vi "estimador de velocidades.vi"() -> (1 "angular speed (rad/s)":dbl, 2 "v_y (cm/s)":dbl, 3 "v_x (cm/s)":dbl)   [LabVIEW 2016]
uses:
  SSL Detection Frame.ctl
  SSL Detection Robot.ctl
  SSL Detection Ball.ctl
panel:
  in  "Detection Frame In":T1
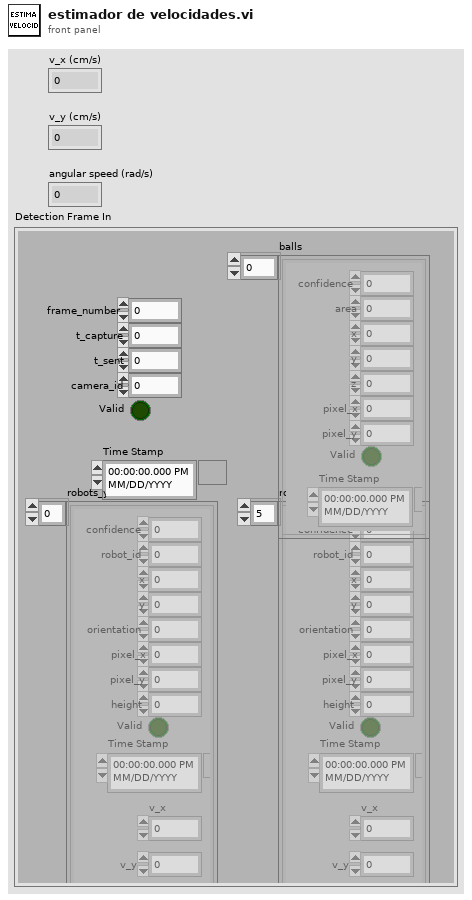
[diagram p1: front panel]
types:
  T1 = typedef "SSL Detection Frame.ctl" = cluster{"frame_number":u32, "t_capture":dbl, "t_sent":dbl, "camera_id":u32, "robots_yellow":T2[], "robots_blue":T2[], "balls":T3[], "Valid":bool, "Time Stamp":timestamp}
  T2 = typedef "SSL Detection Robot.ctl" = cluster{"x":dbl, "robot_id":u32, "confidence":sgl, "y":sgl, "orientation":sgl, "pixel_x":sgl, "pixel_y":sgl, "height":sgl, "Valid":bool, "Time Stamp":timestamp, "v_x":dbl, "v_y":dbl, "v_ang":dbl}
  T3 = typedef "SSL Detection Ball.ctl" = cluster{"x":sgl, "area":u32, "confidence":sgl, "y":sgl, "z":sgl, "pixel_x":sgl, "pixel_y":sgl, "Valid":bool, "Time Stamp":timestamp}
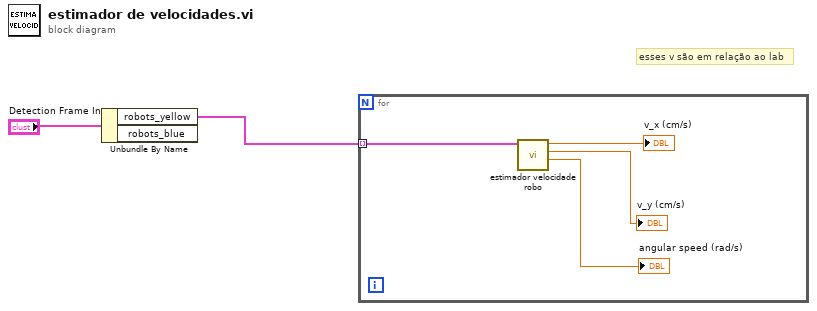
[diagram p0: block diagram]
diagram:
  # "esses v são em relação ao lab"
  n1 = Unbundle By Name("Detection Frame In") -> ("robots_yellow"=w1:T2[])  [unwired: 1 out]
  n2 = for {
    tunnel: w1 -> [w3] mode=indexing
    n3 = call "estimador velocidade robo.vi"("Detection Robot"=w3) -> ("angular speed (rad/s)"=→"angular speed (rad/s)":dbl, "v_y (cm/s)"=→"v_y (cm/s)":dbl, "v_x (cm/s)"=→"v_x (cm/s)":dbl)  [unwired: 8 in]
  }
